vi "CANOpen_Get Section References by GUID for SDOs.vi"(7 "Nodes":T2[](array[typedef]) {"NMT"."Node init static SDO state" items=["start remote node"=1, "enter pre-operational"=128]; "NMT"."Node run state" items=["start remote node"=1, "stop remote node"=2, "enter pre-operational"=128, "reset node"=129, "reset communication"=130]; "Dynamic SDOs"."Sub-Index (0)" format="%.0x"; "Dynamic SDOs"."Object Index" format="%.0x"; "Dynamic SDOs"."Block Data" format="%.0x"; "RPDOs"."PDO Channel" items=["PDO 1", "PDO 2", "PDO 3", "PDO 4"]; "RPDOs"."Parameters"."Bit Offset" max=8 step=1; "RPDOs"."Parameters"."Byte Offset" max=8 step=1; "TPDOs"."PDO Channel" items=["PDO 1", "PDO 2", "PDO 3", "PDO 4"]; "TPDOs"."Parameters"."Bit Offset" max=8 step=1; "TPDOs"."Parameters"."Byte Offset" max=8 step=1; "SDOs"."Sub-Index (0)" format="%.0x"; "SDOs"."Object Index" format="%.0x"; "SDOs"."Block Data" format="%.0x"}, 8 "error in (no error)":errorcluster, 9 "Node Refs":T1[](array[typedef]) format="%.0x", 11 "Device Ref":T1 format="%.0x") -> (0 "error out":errorcluster, 2 "Data References":T11 {"HW Dyn Read"."Resp Chan."."Chan Refs" format="%.0x"; "HW Dyn Read"."Req Chan."."Chan Refs" format="%.0x"; "HW Dyn Write"."Resp Chan."."Chan Refs" format="%.0x"; "HW Dyn Write"."Req Chan."."Chan Refs" format="%.0x"; "List SDO"."Resp Chan."."Chan Refs" format="%.0x"; "List SDO"."Req Chan."."Chan Refs" format="%.0x"}, 3 "Device Ref out":T1=18446744073709551615 format="%.0x")   [LabVIEW 2021, in "CANOpen Addon Engine.lvlib"]
uses:
  CANOpen Addon Engine.lvlib
  <vilib>/NI VeriStand/Custom Device API/Custom Device Item Ref.ctl
  CANOpen_VS SDOs Data Refs.ctl
  <vilib>/NI VeriStand/Custom Device API/Data Reference.ctl
  Async VIs/CANOpen_Main/SubVIs/CanOpen_SDO Dynamic queue.ctl
  Shared/CANOpen_SDO queue W data.ctl
  Shared/CANOpen_SDO queue mode.ctl
  Shared/CANOpen_PDO Data Type in queue.ctl
  CANOpen_Node Message Settings.ctl
  Shared/CANOpen_PDO Settings.ctl
  Shared/CANOpen_PDO Parameter Settings.ctl
  Shared/CANOpen_PDO Data Type.ctl
  System Explorer/SubVIs/CANopen Byte Order.ctl
  Shared/CANOpen_SDO Settings.ctl
  CANOpen_NMT Settings.ctl
  Async VIs/CANOpen_Main/SubVIs/CanOpen_NMT_Config.ctl
  Async VIs/CANOpen_Main/SubVIs/CanOpen_NMT_Static detect.ctl
  Shared/CANOpen Addon GUID Lookup Global.vi
  <vilib>/NI VeriStand/Custom Device Tools/Custom Device Utility Library/NI VeriStand - Search for Item by GUID.vi
  <vilib>/NI VeriStand/Custom Device API/NI VeriStand - Get Channel Data Reference.vi
  <vilib>/NI VeriStand/Custom Device Tools/Custom Device Utility Library/NI VeriStand - Search for All Items by GUID.vi
  <vilib>/NI VeriStand/Custom Device API/Custom Device API.lvlib
  <vilib>/NI VeriStand/Custom Device Tools/Custom Device Utility Library/Custom Device Utility Library.lvlib
  Shared/CANOpen Addon Shared.lvlib
  System Explorer/CANOpen Addon System Explorer.lvlib
panel:
  # "LSB"
  # "MSB"
  # "LSB"
  # "MSB"
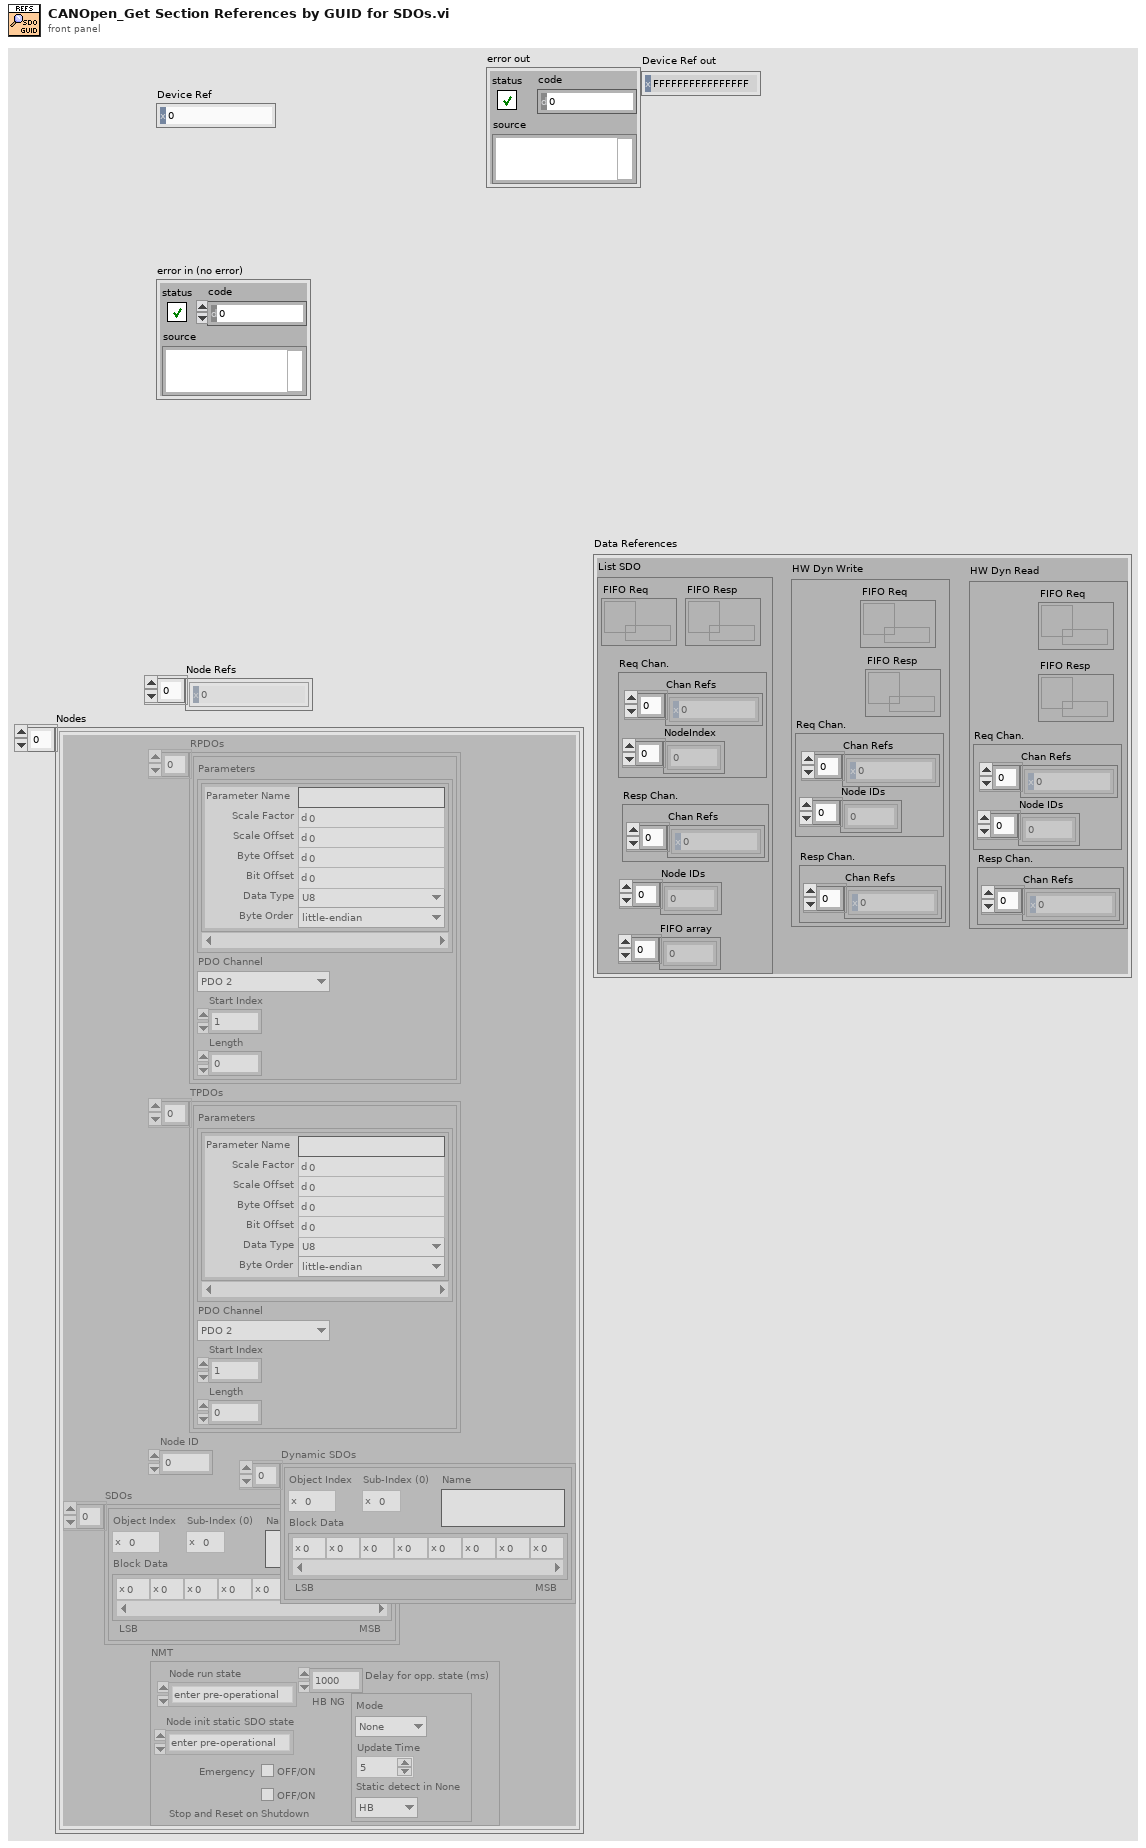
[diagram p1: front panel]
types:
  T1 = typedef "Custom Device API.lvlib/Custom Device Item Ref.ctl" = u64
  T2 = typedef "CANOpen Addon Engine.lvlib/CANOpen_Node Message Settings.ctl" = cluster{"RPDOs":T3[], "TPDOs":T3[], "Node ID":u8, "SDOs":T7[], "Dynamic SDOs":T7[], "NMT":T8}
  T3 = typedef "CANOpen Addon Shared.lvlib/CANOpen_PDO Settings.ctl" = cluster{"Parameters":T4[], "PDO Channel":u8, "Start Index":u32, "Length":u32}
  T4 = typedef "CANOpen Addon Shared.lvlib/CANOpen_PDO Parameter Settings.ctl" = cluster{"Parameter Name":string, "Scale Factor":dbl, "Scale Offset":dbl, "Byte Offset":u8, "Bit Offset":u8, "Data Type":T5, "Byte Order":T6}
  T5 = typedef "CANOpen Addon Shared.lvlib/CANOpen_PDO Data Type.ctl" = enum16{"U8", "U16", "U32", "I8", "I16", "I32", "Single", "Double", "Boolean"}
  T6 = typedef "CANOpen Addon System Explorer.lvlib/CANopen Byte Order.ctl" = enum16{"big-endian network order", "little-endian"}
  T7 = typedef "CANOpen Addon Shared.lvlib/CANOpen_SDO Settings.ctl" = cluster{"Object Index":u16, "Sub-Index (0)":u8, "Block Data":u8[], "Name":string}
  T8 = typedef "CANOpen Addon Engine.lvlib/CANOpen_NMT Settings.ctl" = cluster{"Node run state":u16, "Emergency":bool, "HB NG":T9, "Delay for opp. state (ms)":dbl, "Node init static SDO state":u16, "Stop and Reset on Shutdown":bool}
  T9 = typedef "CANOpen Addon Engine.lvlib/CanOpen_NMT_Config.ctl" = cluster{"Mode":T10, "Update Time":u16, "Static detect in None":T10}
  T10 = typedef "CANOpen Addon Engine.lvlib/CanOpen_NMT_Static detect.ctl" = enum16{"None", "HB", "NG"}
  T11 = typedef "CANOpen Addon Engine.lvlib/CANOpen_VS SDOs Data Refs.ctl" = cluster{"List SDO":cluster{"FIFO Req":refnum<k33>, "Req Chan.":cluster{"Chan Refs":T12[], "NodeIndex":dbl[]}, "FIFO Resp":refnum<k33>, "Resp Chan.":cluster{"Chan Refs":T12[]}, "Node IDs":u8[], "FIFO array":dbl[]}, "HW Dyn Write":cluster{"FIFO Req":refnum<k33>, "FIFO Resp":refnum<k33>, "Req Chan.":cluster{"Chan Refs":T12[], "Node IDs":u8[]}, "Resp Chan.":cluster{"Chan Refs":T12[]}}, "HW Dyn Read":cluster{"FIFO Req":refnum<k33>, "FIFO Resp":refnum<k33>, "Req Chan.":cluster{"Chan Refs":T12[], "Node IDs":u8[]}, "Resp Chan.":cluster{"Chan Refs":T12[]}}}
  T12 = typedef "Custom Device API.lvlib/Data Reference.ctl" = i32
  T13 = cluster{"read mode":enum16{"polling", "blocking"}, "write mode":enum16{"polling", "blocking"}}
  T14 = typedef "CANOpen Addon Engine.lvlib/CanOpen_SDO Dynamic queue.ctl" = cluster{"Node ID":u8, "Data":T15}
  T15 = typedef "CANOpen Addon Shared.lvlib/CANOpen_SDO queue W data.ctl" = cluster{"Object Index":u16, "Object Sub-Index (0)":u8, "Mode":T16, "Data Type":T17, "Value":dbl, "Status code":dbl, "Byte Order":enum16{"big-endian, network order", "little-endian"}}
  T16 = typedef "CANOpen Addon Shared.lvlib/CANOpen_SDO queue mode.ctl" = enum16{"WRITE write", "WRITE response", "READ write", "READ response"}
  T17 = typedef "CANOpen Addon Shared.lvlib/CANOpen_PDO Data Type in queue.ctl" = enum16{"U8", "U16", "U32", "I8", "I16", "I32", "Single", "Double"}
  T18 = typedef "Custom Device API.lvlib/Custom Device Item Info.ctl" = cluster{"Name":string, "Is Channel":bool, "GUID":string, "Is Waveform":bool}
  T19 = typedef "CANOpen Addon Engine.lvlib/CanOpen_Main Node Ids.ctl" = u8[]
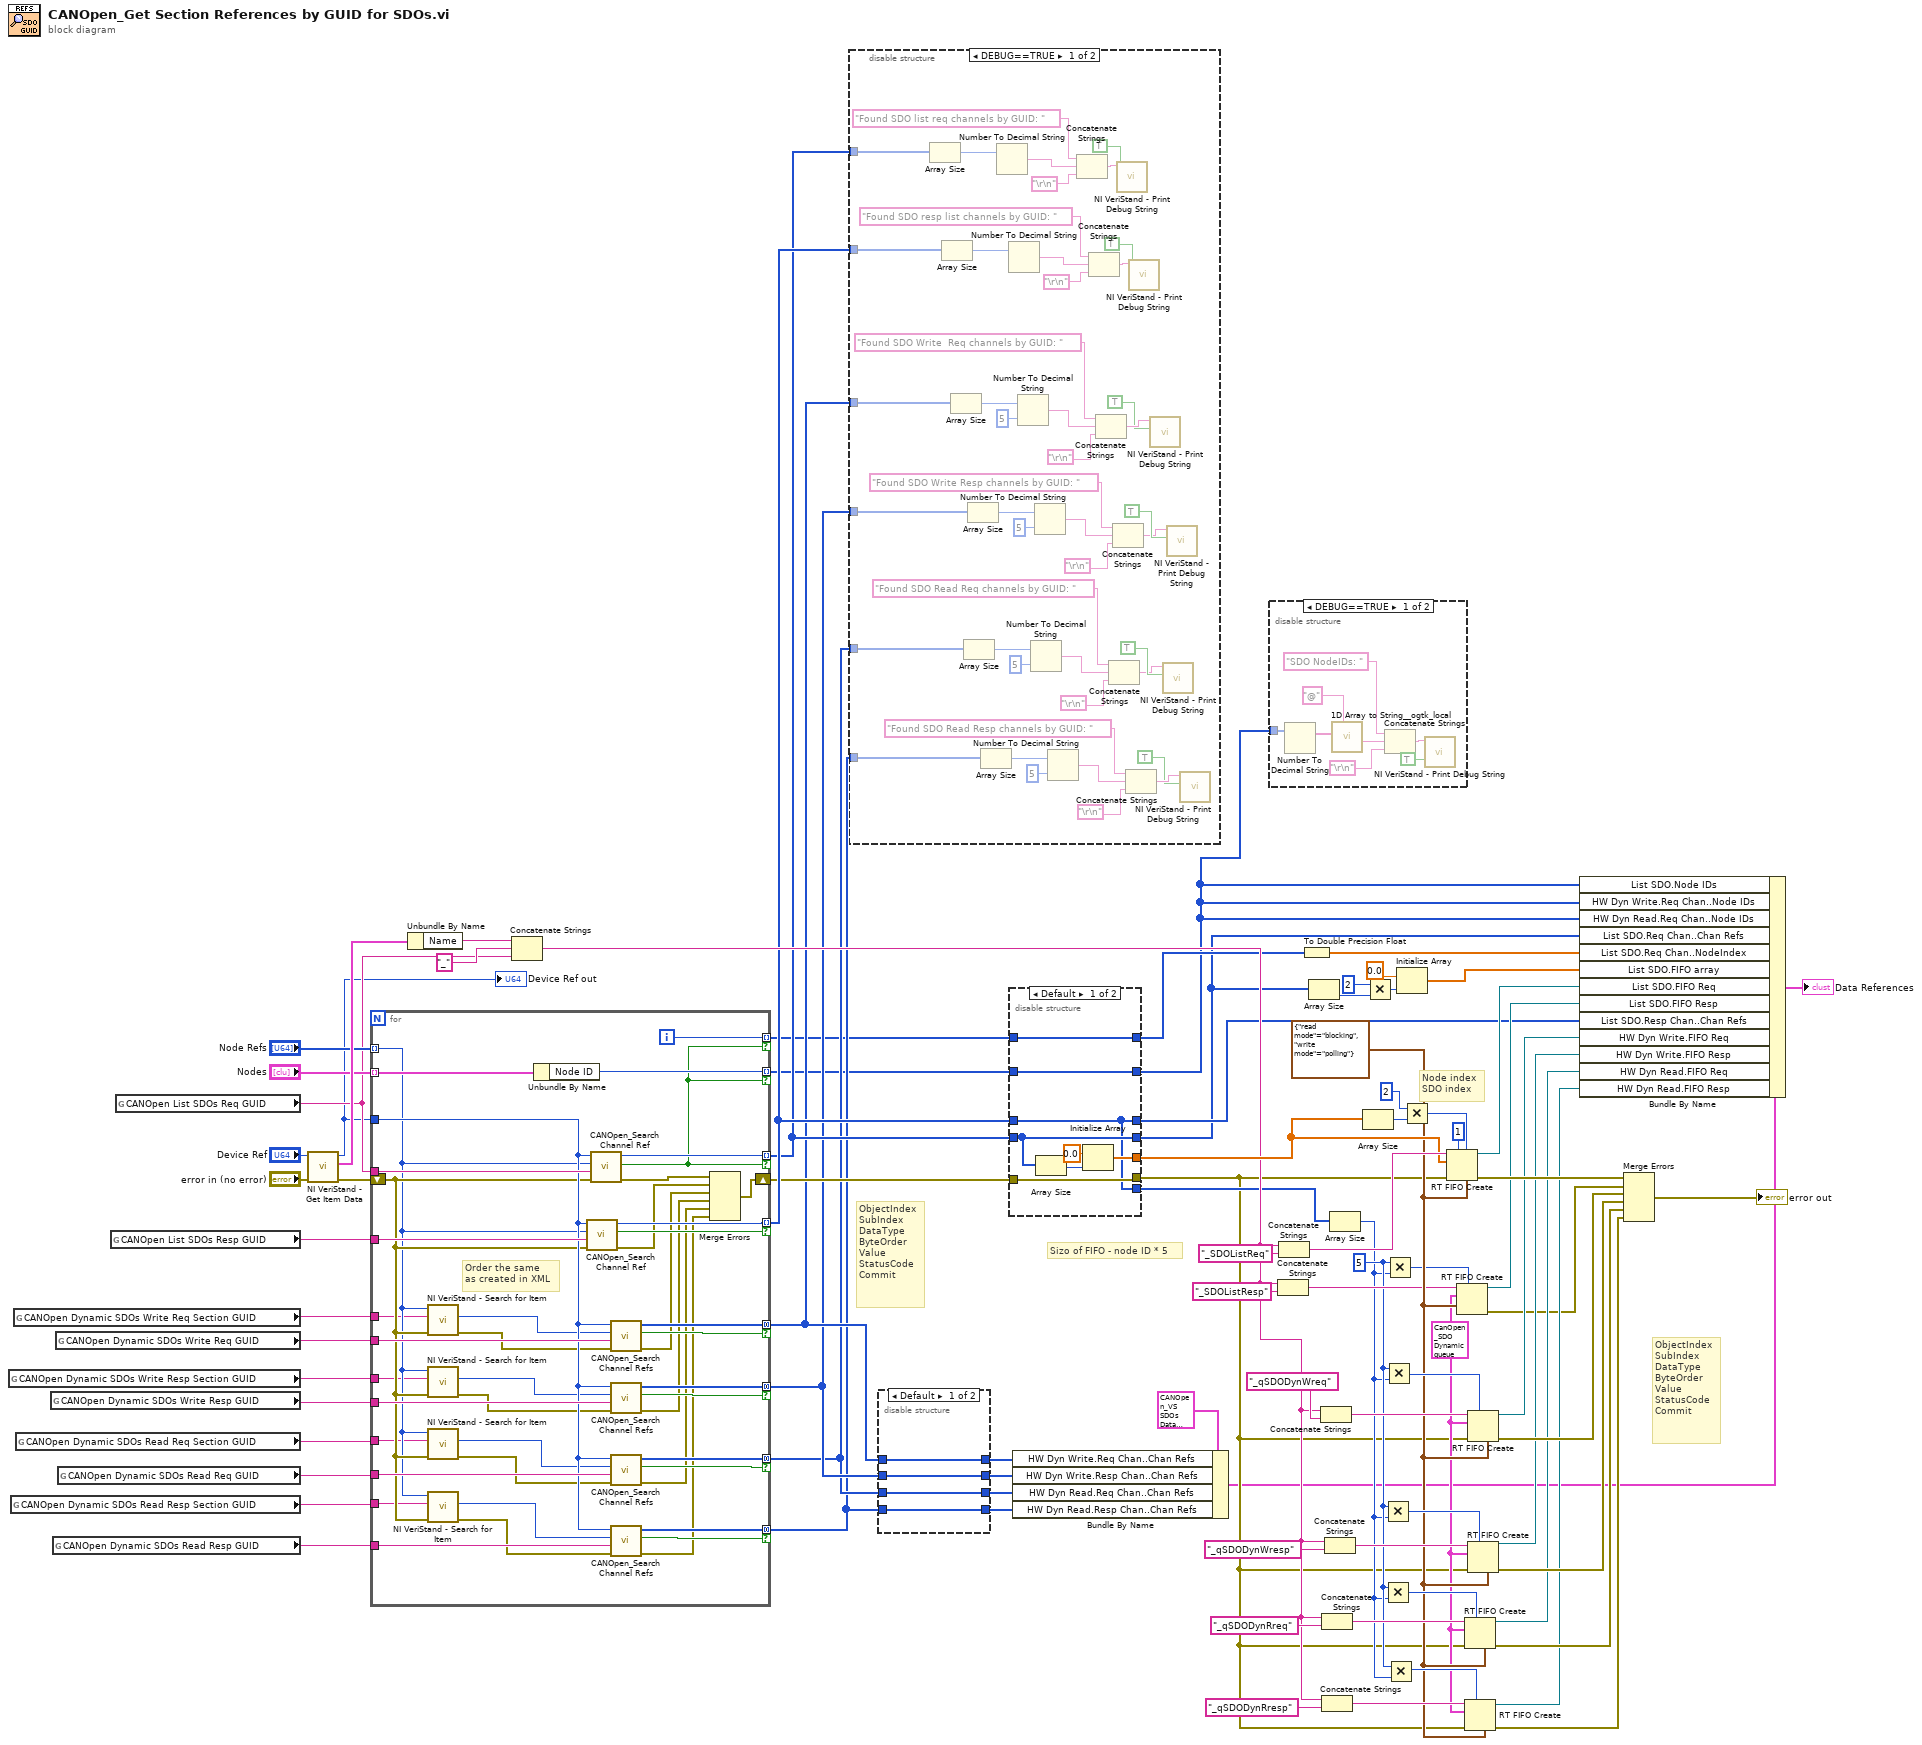
[diagram p0: block diagram]
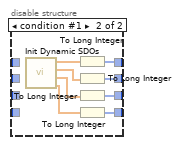
[diagram p2: hidden frame]
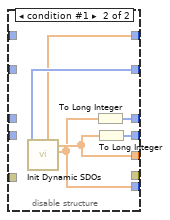
[diagram p3: hidden frame]
diagram:
  w35 = 5 ("x")
  w41 = T13 {"read mode"=enum."blocking", "write mode"=enum."polling"} ("r/w modes (polling,polling)")
  w38 = T14 {"Node ID"=0, "Data"={"Object Index"=0, "Object Sub-Index (0)"=0, "Mode"=enum."WRITE write", "Data Type"=enum."U8", "Value"=0.0, "Status code"=0.0, "Byte Order"=enum."little-endian"}} ("element")
  # "ObjectIndex\nSubIndex\nDataType\nByteOrder\nValue\nStatusCode\nCommit"
  # "ObjectIndex\nSubIndex\nDataType\nByteOrder\nValue\nStatusCode\nCommit"
  # "Sizo of FIFO - node ID * 5"
  # "Node index\nSDO index"
  n1 = global read "CANOpen Addon GUID Lookup Global.vi" "CANOpen Dynamic SDOs Write Resp Section GUID"() -> (w10:string)
  n2 = global read "CANOpen Addon GUID Lookup Global.vi" "CANOpen Dynamic SDOs Read Resp Section GUID"() -> (w8:string)
  n3 = global read "CANOpen Addon GUID Lookup Global.vi" "CANOpen Dynamic SDOs Write Req Section GUID"() -> (w11:string)
  n4 = global read "CANOpen Addon GUID Lookup Global.vi" "CANOpen Dynamic SDOs Read Req Section GUID"() -> (w9:string)
  n5 = global read "CANOpen Addon GUID Lookup Global.vi" "CANOpen Dynamic SDOs Write Resp GUID"() -> (w63:string)
  n6 = global read "CANOpen Addon GUID Lookup Global.vi" "CANOpen Dynamic SDOs Read Resp GUID"() -> (w53:string)
  n7 = global read "CANOpen Addon GUID Lookup Global.vi" "CANOpen Dynamic SDOs Write Req GUID"() -> (w80:string)
  n8 = global read "CANOpen Addon GUID Lookup Global.vi" "CANOpen Dynamic SDOs Read Req GUID"() -> (w54:string)
  n9 = global read "CANOpen Addon GUID Lookup Global.vi" "CANOpen List SDOs Resp GUID"() -> (w36:string)
  n10 = global read "CANOpen Addon GUID Lookup Global.vi" "CANOpen List SDOs Req GUID"() -> (w44:string)
  n11 = call <vilib>:"NI VeriStand - Get Item Data.vi"("error in (no error)"="error in (no error)", "Item Ref in"="Device Ref") -> ("error out"=w82:errorcluster, "Item Info"=w87:T18, "Item Ref out"=w31:T1)  [unwired: 6 in, 1 out]
  "Device Ref out" <- w31
  n12 = for {
    tunnel: w44 -> [w130]
    tunnel: "Node Refs" -> [w92] mode=indexing
    shift-right: [w104] -> w25
    shift-left: w82 -> [w101]
    tunnel: w80 -> [w123]
    tunnel: [w127] -> w24 mode=indexing if=w102
    tunnel: [w116] -> w22 mode=concatenating if=w118
    tunnel: "Nodes" -> [w129] mode=indexing
    tunnel: [w128] -> w15 mode=indexing if=w102
    tunnel: w63 -> [w122]
    tunnel: [w115] -> w21 mode=concatenating if=w117
    tunnel: w54 -> [w121]
    tunnel: w53 -> [w120]
    tunnel: [w114] -> w19 mode=concatenating if=w113
    tunnel: [w112] -> w17 mode=concatenating if=w111
    tunnel: w36 -> [w126]
    tunnel: [w124] -> w26 mode=indexing if=w125
    tunnel: w31 -> [w119]
    tunnel: [w103] -> w13 mode=indexing if=w102
    tunnel: w11 -> [w91]
    tunnel: w10 -> [w90]
    tunnel: w9 -> [w89]
    tunnel: w8 -> [w88]
    i -> [w103]
    # "Order the same\nas created in XML"
    n13 = call-poly <vilib>:"NI VeriStand - Search for Item.vi"("error in"=w101, "Item GUID"=w91, "Section Ref in"=w92) -> ("error out"=w100:errorcluster, "Item Ref"=w96:T1)  [unwired: 5 in, 2 out]
    n14 = call-poly <vilib>:"NI VeriStand - Search for Item.vi"("error in"=w101, "Item GUID"=w90, "Section Ref in"=w92) -> ("error out"=w99:errorcluster, "Item Ref"=w95:T1)  [unwired: 5 in, 2 out]
    n15 = call-poly <vilib>:"NI VeriStand - Search for Item.vi"("error in"=w101, "Item GUID"=w89, "Section Ref in"=w92) -> ("error out"=w98:errorcluster, "Item Ref"=w94:T1)  [unwired: 5 in, 2 out]
    n16 = call-poly <vilib>:"NI VeriStand - Search for Item.vi"("error in"=w101, "Item GUID"=w88, "Section Ref in"=w92) -> ("error out"=w97:errorcluster, "Item Ref"=w93:T1)  [unwired: 5 in, 2 out]
    n17 = Unbundle By Name(w129) -> ("Node ID"=w128:u8)
    n18 = call "CANOpen_Search Channel Ref.vi"("error in (no error)"=w101, "GUID"=w126, "Section Ref in"=w92, "Device Ref"=w119) -> ("error out"=w109:errorcluster, "Found"=w125:bool, "Channel Data Reference"=w124:T12)  [unwired: 5 in]
    n19 = call "CANOpen_Search Channel Ref.vi"("error in (no error)"=w101, "GUID"=w130, "Section Ref in"=w92, "Device Ref"=w119) -> ("error out"=w110:errorcluster, "Found"=w102:bool, "Channel Data Reference"=w127:T12)  [unwired: 5 in]
    n20 = call "CANOpen_Search Channel Refs.vi"("error in (no error)"=w100, "GUID"=w123, "Section Ref in"=w96, "Device Ref"=w119) -> ("error out"=w108:errorcluster, "Found"=w118:bool, "Channel Data References"=w116:T12[])  [unwired: 5 in]
    n21 = call "CANOpen_Search Channel Refs.vi"("error in (no error)"=w99, "GUID"=w122, "Section Ref in"=w95, "Device Ref"=w119) -> ("error out"=w107:errorcluster, "Found"=w117:bool, "Channel Data References"=w115:T12[])  [unwired: 5 in]
    n22 = call "CANOpen_Search Channel Refs.vi"("error in (no error)"=w98, "GUID"=w121, "Section Ref in"=w94, "Device Ref"=w119) -> ("error out"=w106:errorcluster, "Found"=w113:bool, "Channel Data References"=w114:T12[])  [unwired: 5 in]
    n23 = call "CANOpen_Search Channel Refs.vi"("error in (no error)"=w97, "GUID"=w120, "Section Ref in"=w93, "Device Ref"=w119) -> ("error out"=w105:errorcluster, "Found"=w111:bool, "Channel Data References"=w112:T12[])  [unwired: 5 in]
    n24 = Merge Errors(w110, w109, w108, w107, w106, w105) -> (w104:errorcluster)
  }
  n25 = Unbundle By Name(w87) -> ("Name"=w84:string)
  n26 = Concatenate Strings(w84, "_" ("string"), w44) -> (w42:string)
  n27 = disable-structure shown="DEBUG==TRUE" {
    disable-tunnel: w24 -> [w174 _]
    disable-tunnel: w22 -> [w169 _]
    disable-tunnel: w21 -> [w154 _]
    disable-tunnel: w19 -> [w139 _]
    disable-tunnel: w17 -> [w138 _]
    disable-tunnel: w26 -> [w131 _]
    frame condition #0 {
      n28 = Array Size(array=w174) -> (size(s)=w173:i32)
      n29 = Array Size(array=w131) -> (size(s)=w134:i32)
      n30 = Array Size(array=w169) -> (size(s)=w170:i32)
      n31 = Array Size(array=w139) -> (size(s)=w140:i32)
      n32 = Array Size(array=w154) -> (size(s)=w155:i32)
      n33 = Array Size(array=w138) -> (size(s)=w153:i32)
      n34 = Number To Decimal String(number=w173) -> (decimal integer string=w172:string)  [unwired: 1 in]
      n35 = Number To Decimal String(number=w134) -> (decimal integer string=w135:string)  [unwired: 1 in]
      n36 = Number To Decimal String(number=w170, width (-)=i16 5) -> (decimal integer string=w166:string)
      n37 = Number To Decimal String(number=w140, width (-)=i16 5) -> (decimal integer string=w143:string)
      n38 = Number To Decimal String(number=w155, width (-)=i16 5) -> (decimal integer string=w158:string)
      n39 = Number To Decimal String(number=w153, width (-)=i16 5) -> (decimal integer string=w150:string)
      n40 = Concatenate Strings("Found SDO list req channels by GUID: " ("string"), w172, "\r\n") -> (w176:string)
      n41 = Concatenate Strings("Found SDO resp list channels by GUID: " ("string"), w135, "\r\n") -> (w132:string)
      n42 = Concatenate Strings("Found SDO Write  Req channels by GUID: " ("string"), w166, "\r\n") -> (w164:string)
      n43 = Concatenate Strings("Found SDO Read Req channels by GUID: " ("string"), w143, "\r\n") -> (w145:string)
      n44 = Concatenate Strings("Found SDO Write Resp channels by GUID: " ("string"), w158, "\r\n") -> (w160:string)
      n45 = call <vilib>:"NI VeriStand - Print Debug String.vi"("Add to log file? (F)"=TRUE ("Add to log file? (T)"), "Message"=w176) -> ()  [unwired: 9 in, 1 out]
      n46 = Concatenate Strings("Found SDO Read Resp channels by GUID: " ("string"), w150, "\r\n") -> (w148:string)
      n47 = call <vilib>:"NI VeriStand - Print Debug String.vi"("Add to log file? (F)"=TRUE ("Add to log file? (T)"), "Message"=w132) -> ()  [unwired: 9 in, 1 out]
      n48 = call <vilib>:"NI VeriStand - Print Debug String.vi"("Add to log file? (F)"=TRUE ("Add to log file? (T)"), "Message"=w164) -> ()  [unwired: 9 in, 1 out]
      n49 = call <vilib>:"NI VeriStand - Print Debug String.vi"("Add to log file? (F)"=TRUE ("Add to log file? (T)"), "Message"=w145) -> ()  [unwired: 9 in, 1 out]
      n50 = call <vilib>:"NI VeriStand - Print Debug String.vi"("Add to log file? (F)"=TRUE ("Add to log file? (T)"), "Message"=w160) -> ()  [unwired: 9 in, 1 out]
      n51 = call <vilib>:"NI VeriStand - Print Debug String.vi"("Add to log file? (F)"=TRUE ("Add to log file? (T)"), "Message"=w148) -> ()  [unwired: 9 in, 1 out]
    }
    frame condition #1 (active) {
    }
  }
  n52 = disable-structure shown="Default" {
    disable-tunnel: [w177 w181] -> w23
    disable-tunnel: w22 -> [w177 _]
    disable-tunnel: w21 -> [w180 _]
    disable-tunnel: [w180 w187] -> w20
    disable-tunnel: w19 -> [w179 _]
    disable-tunnel: [w179 w184] -> w18
    disable-tunnel: w17 -> [w178 _]
    disable-tunnel: [w178 w182] -> w16
    frame condition #0 (active) {
    }
    frame condition #1 {
      n53 = call "Init Dynamic SDOs.vi"() -> ("Resp Dyn Read"=w183:dbl[], "Req Dyn Read"=w185:dbl[], "Resp Dyn Write"=w186:dbl[], "Req Dyn Write"=w188:dbl[])  [unwired: 4 in, 4 out]
      n54 = To Long Integer(number=w188) -> (32bit integer=w181:i32[])
      n55 = To Long Integer(number=w186) -> (32bit integer=w187:i32[])
      n56 = To Long Integer(number=w185) -> (32bit integer=w184:i32[])
      n57 = To Long Integer(number=w183) -> (32bit integer=w182:i32[])
    }
  }
  n58 = disable-structure shown="Default" {
    disable-tunnel: [w196 _] -> w29
    disable-tunnel: [w195 w201] -> w2
    disable-tunnel: [w192 w202] -> w62
    disable-tunnel: w24 -> [w195 _]
    disable-tunnel: w25 -> [w196 _]
    disable-tunnel: [w191 w200] -> w33
    disable-tunnel: w26 -> [w191 _]
    disable-tunnel: [w191 w199] -> w32
    disable-tunnel: [w190 w198] -> w12
    disable-tunnel: w15 -> [w190 _]
    disable-tunnel: [w189 w197] -> w14
    disable-tunnel: w13 -> [w189 _]
    frame condition #0 (active) {
      n59 = Array Size(array=w195) -> (size(s)=w194:i32)
      n60 = Initialize Array(0.0 ("element"), w194) -> (w192:dbl[])
    }
    frame condition #1 {
      n61 = call "Init Dynamic SDOs.vi"() -> ("SDO Node index"=w197:dbl[], "Resp List SDO"=w200:dbl[], "Req List SDO"=w202:dbl[], "Node Ids"=w198:T19)  [unwired: 4 in, 4 out]
      n62 = To Long Integer(number=w200) -> (32bit integer=w199:i32[])
      n63 = To Long Integer(number=w202) -> (32bit integer=w201:i32[])
    }
  }
  n64 = Bundle By Name(cluster=T11 {"List SDO"={"FIFO Req"=refnum, "Req Chan."={"Chan Refs"=[], "NodeIndex"=[]}, "FIFO Resp"=refnum, "Resp Chan."={"Chan Refs"=[]}, "Node IDs"=[], "FIFO array"=[]}, "HW Dyn Write"={"FIFO Req"=refnum, "FIFO Resp"=refnum, "Req Chan."={"Chan Refs"=[], "Node IDs"=[]}, "Resp Chan."={"Chan Refs"=[]}}, "HW Dyn Read"={"FIFO Req"=refnum, "FIFO Resp"=refnum, "Req Chan."={"Chan Refs"=[], "Node IDs"=[]}, "Resp Chan."={"Chan Refs"=[]}}} ("Data References"), "HW Dyn Write.Req Chan..Chan Refs"=w23, "HW Dyn Write.Resp Chan..Chan Refs"=w20, "HW Dyn Read.Req Chan..Chan Refs"=w18, "HW Dyn Read.Resp Chan..Chan Refs"=w16) -> (w27:T11)
  n65 = disable-structure shown="DEBUG==TRUE" {
    disable-tunnel: w12 -> [w210 _]
    frame condition #0 {
      n66 = Number To Decimal String(number=w210) -> (decimal integer string=w209:string[])  [unwired: 1 in]
      n67 = call "1D Array to String__ogtk_local.vi"("delimiter (Tab)"="@", "Array of Strings"=w209) -> ("delimited string"=w207:string)  [unwired: 9 in]
      n68 = Concatenate Strings("SDO NodeIDs: " ("string"), w207, "\r\n") -> (w206:string)
      n69 = call <vilib>:"NI VeriStand - Print Debug String.vi"("Add to log file? (F)"=TRUE ("Add to log file? (T)"), "Message"=w206) -> ()  [unwired: 9 in, 1 out]
    }
    frame condition #1 (active) {
    }
  }
  n70 = Concatenate Strings(w42, "_SDOListResp" ("string")) -> (w40:string)
  n71 = Concatenate Strings(w42, "_SDOListReq" ("string")) -> (w75:string)
  n72 = To Double Precision Float(number=w14) -> (double precision float=w7:dbl[])
  n73 = Array Size(array=w2) -> (size(s)=w3:i32)
  n74 = Concatenate Strings(w42, "_qSDODynWreq" ("name (unnamed)")) -> (w67:string)
  n75 = Concatenate Strings(w42, "_qSDODynRreq" ("name (unnamed)")) -> (w65:string)
  n76 = Concatenate Strings(w42, "_qSDODynRresp" ("name (unnamed)")) -> (w58:string)
  n77 = Concatenate Strings(w42, "_qSDODynWresp" ("name (unnamed)")) -> (w66:string)
  n78 = Array Size(array=w33) -> (size(s)=w30:i32)
  n79 = Array Size(array=w62) -> (size(s)=w74:i32)
  n80 = Multiply(x=2, y=w3) -> (x*y=w4:i32)
  n81 = Multiply(x=w35, y=w30) -> (x*y=w51:i32)
  n82 = Multiply(x=w35, y=w30) -> (x*y=w50:i32)
  n83 = Multiply(x=w35, y=w30) -> (x*y=w52:i32)
  n84 = Multiply(x=w35, y=w30) -> (x*y=w34:i32)
  n85 = Multiply(x=w35, y=w30) -> (x*y=w49:i32)
  n86 = Initialize Array(0.0 ("Numeric"), w4) -> (w1:dbl[])
  n87 = Multiply(x=2, y=w74) -> (x*y=w72:i32)
  n88 = RT FIFO Create(0:w75, 1:w62, 3:w29, 4:u32 1 ("size (10)"), 6:w72, 7:w41) -> (8:w78:refnum<k33>, 11:w71:errorcluster)  [unwired: 2 in, 1 out]
  n89 = RT FIFO Create(0:w40, 1:w38, 4:w34, 7:w41) -> (8:w39:refnum<k33>, 11:w37:errorcluster)  [unwired: 4 in, 1 out]
  n90 = RT FIFO Create(0:w65, 1:w38, 3:w29, 4:w50, 7:w41) -> (8:w46:refnum<k33>, 11:w56:errorcluster)  [unwired: 3 in, 1 out]
  n91 = RT FIFO Create(0:w58, 1:w38, 3:w29, 4:w49, 7:w41) -> (8:w45:refnum<k33>, 11:w55:errorcluster)  [unwired: 3 in, 1 out]
  n92 = RT FIFO Create(0:w67, 1:w38, 3:w29, 4:w52, 7:w41) -> (8:w48:refnum<k33>, 11:w60:errorcluster)  [unwired: 3 in, 1 out]
  n93 = RT FIFO Create(0:w66, 1:w38, 3:w29, 4:w51, 7:w41) -> (8:w47:refnum<k33>, 11:w57:errorcluster)  [unwired: 3 in, 1 out]
  n94 = Bundle By Name(cluster=w27, "List SDO.Node IDs"=w12, "HW Dyn Write.Req Chan..Node IDs"=w12, "HW Dyn Read.Req Chan..Node IDs"=w12, "List SDO.Req Chan..Chan Refs"=w2, "List SDO.Req Chan..NodeIndex"=w7, "List SDO.FIFO array"=w1, "List SDO.FIFO Req"=w78, "List SDO.FIFO Resp"=w39, "List SDO.Resp Chan..Chan Refs"=w32, "HW Dyn Write.FIFO Req"=w48, "HW Dyn Write.FIFO Resp"=w47, "HW Dyn Read.FIFO Req"=w46, "HW Dyn Read.FIFO Resp"=w45) -> (→"Data References":T11)
  n95 = Merge Errors(w71, w37, w60, w57, w56, w55) -> (→"error out":errorcluster)
